vi "uActor_SendReservedMsg.vi"(8 "error in (no error)":errorcluster, 10 "Msg":refnum<class "uMsg.lvclass">, 11 "uActor Transport":refnum<class "uTransport_uActor.lvclass">) -> (0 "error out":errorcluster)   [LabVIEW 2021, in "uFramework.lvlib" / "uActor.lvclass"]
doc: "Special method to send architectural critical messages."
uses:
  uTransport_uActor/uTransport_uActor.lvclass
  uMsg/uMsg.lvclass
  uMsg/uMsg.lvclass/uMsg.ctl
  uTransport_uActor/uTransport_uActor.lvclass/uTransport_uActor.ctl
  uActor.lvclass
  uActor.lvclass/uActor.ctl
  Bin/uData.lvlibp/uData.lvclass
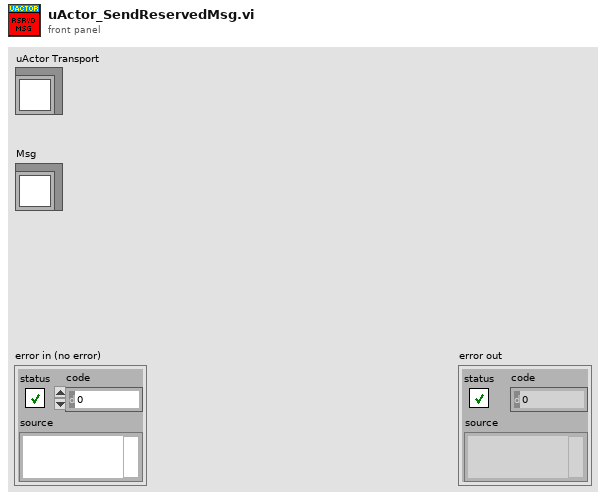
[diagram p1: front panel]
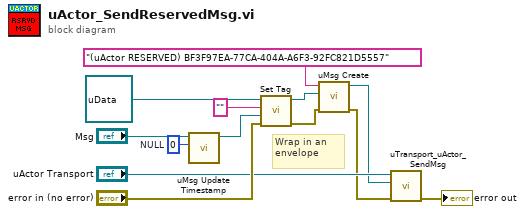
[diagram p0: block diagram]
diagram:
  w10 = u32 0  # NULL
  # "Wrap in an envelope"
  n1 = call "uMsg Update Timestamp.vi"("Timestamp"=w10, "uMsg in"="Msg") -> ("uMsg out"=w4:refnum<class "uMsg.lvclass">)  [unwired: 8 in, 1 out]
  n2 = call "Set Tag.vi"("error in (no error)"="error in (no error)", "Variant"=w4, "tag (case insensitive)"="", "uData in"=refnum<class "uData.lvclass"> refnum) -> ("error out"=w7:errorcluster, "uData out"=w6:refnum<class "uData.lvclass">)  [unwired: 5 in, 1 out]
  n3 = call "uMsg Create.vi"("error in (no error)"=w7, "Payload"=w6, "CMD"="(uActor RESERVED) BF3F97EA-77CA-404A-A6F3-92FC821D5557") -> ("error out"=w1:errorcluster, "uMsg out"=w2:refnum<class "uMsg.lvclass">)  [unwired: 7 in]
  n4 = call "uTransport_uActor_SendMsg.vi"("error in (no error)"=w1, "Msg"=w2, "uTransport_uActor in"="uActor Transport") -> ("error out"=→"error out":errorcluster)  [unwired: 8 in]
